vi "Engine-DI-Calibration.vi"(8 "error in (no error)":errorcluster, 9 "Inj Qtys DI-B":sgl[][](array[numeric]), 10 "Inj Qtys DI-A":sgl[][](array[numeric]), 11 "DCM DSI":refnum<class "DCM-DSI.lvclass">) -> (0 "error out":errorcluster, 3 "DCM DSI":refnum<class "DCM-DSI.lvclass">)   [LabVIEW 2016, in "DSI-RT.lvlib"]
uses:
  DSI-RT.lvlib
  Classes/DCM-DSI/DCM-DSI.lvclass
  Classes/DCM-DSI/Read DI-A Command.vi
  Classes/DCM-DSI/Read DI-B Command.vi
  Classes/DCM-DSI/Read Channels.vi
  Classes/DCM-DSI/Write DI-A Command.vi
  Classes/DCM-DSI/Write DI-B Command.vi
  <vilib>/addons/Software Calibration Management/xSCM/CalPoint.xnode
  <vilib>/addons/Software Calibration Management/xSCM/ni_scm.dll
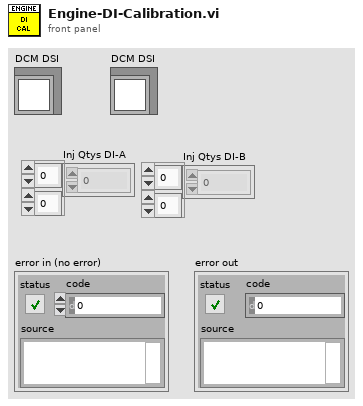
[diagram p1: front panel]
types:
  T1 = typedef "DCM - RT - DI.lvlib/Command.ctl" = cluster{"Mode":T2, "Digital Input":T3, "Default Profile Index":u8, "Cal Freq [Hz]":sgl, "Cal Duration [s]":sgl, "Cal Increment [s]":sgl, "Cal Pulses":u16, "TMP Command Sequence":T4[], "EPT TDC Offset [CAD]":sgl, "EPT Window Start [DBTDC]":sgl, "EPT Window End [DBTDC]":sgl, "EPT Angles":T5[], "EPT Skip Fire":bool, "EPT Skip Index":u8, "EPT Precharge Duration [s]":sgl, "EPT Precharge Profile Index":u8}
  T2 = typedef "DCM - FPGA - DI.lvlib/Mode.ctl" = enum8{"Off", "Direct", "Calibration", "Triggered Multi-Pulse", "Engine Position Tracking"}
  T3 = typedef "DCM - FPGA.lvlib/Digital Channel.ctl" = enum8{"Unused", "User OS", "Diff IO 1", "Diff IO 2", "Diff IO 3", "Diff IO 4", "Diff IO 5", "Diff IO 6", "Diff IO 7", "Diff IO 8", "Aux 1", "Aux 2", "Aux 3", "Aux 4", "Aux 5", "Aux 6", "Aux 7", "Aux 8", "Aux 9", "Aux 10", "Aux 11", "Aux 12", "Aux 13", "Aux 14", "Aux 15", "Aux 16"}
  T4 = typedef "DCM - RT - DI.lvlib/Command Sequence.ctl" = cluster{"Duration [s]":sgl, "Level":bool, "Run/Stop":bool, "Profile Index":u8}
  T5 = typedef "DCM - RT - DI.lvlib/Angle Control.ctl" = cluster{"Enable":bool, "Timing [DBTDC]":sgl, "Duration [s]":sgl, "Profile Index":u8}
  T6 = typedef "DCM-DSI.lvclass/Channel.ctl" = cluster{"Name":string, "Unit":string, "Value":sgl}
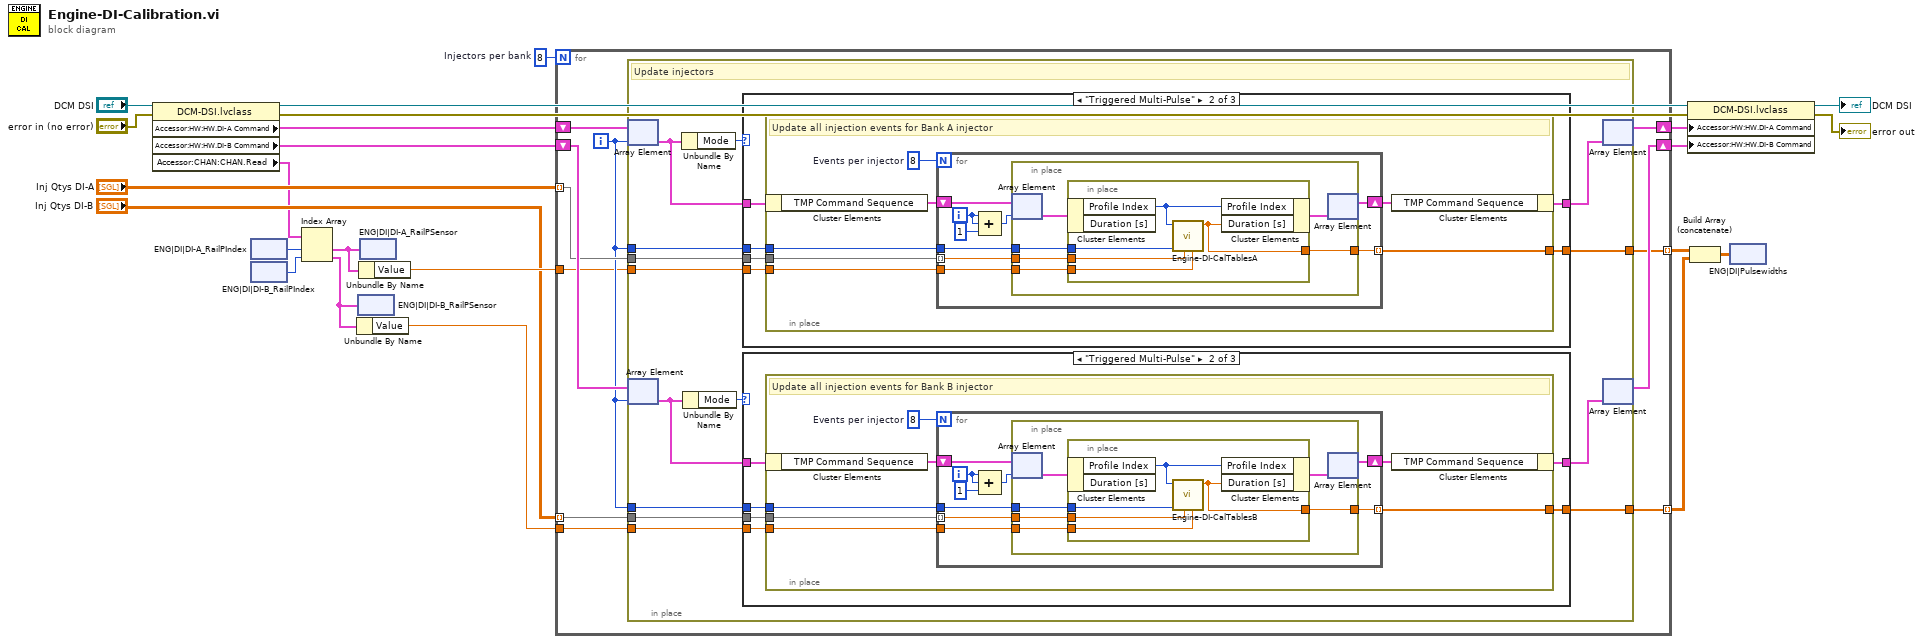
[diagram p0: block diagram]
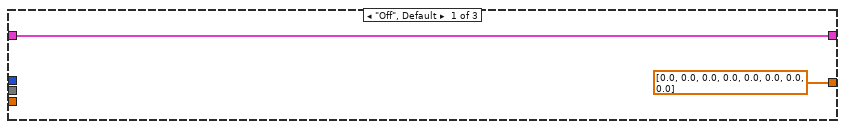
[diagram p2: hidden frame]
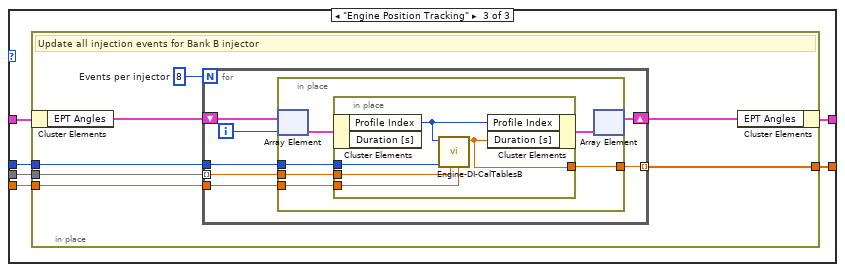
[diagram p3: hidden frame]
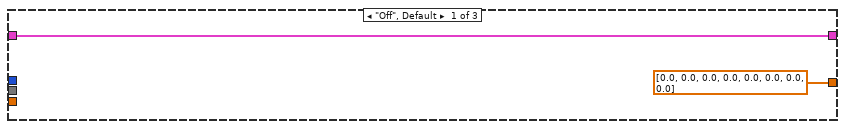
[diagram p4: hidden frame]
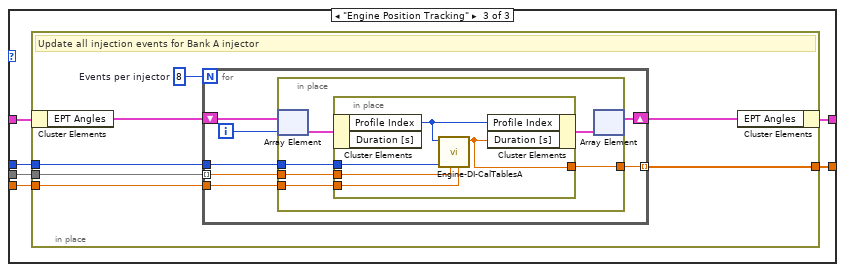
[diagram p5: hidden frame]
diagram:
  w22 = 8  # Injectors per bank
  n1 = property class="DCM-DSI.lvclass"(reference="DCM DSI", error in="error in (no error)") -> (reference out=w18:refnum<class "DCM-DSI.lvclass">, error out=w17:errorcluster, "Accessor:HW:HW.DI-A Command"=w9:T1[], "Accessor:HW:HW.DI-B Command"=w10:T1[], "Accessor:CHAN:CHAN.Read"=w5:T6[])
  n2 = xnode "ENG|DI|DI-A_RailPIndex"() -> ("Value"=w2:i32)
  n3 = xnode "ENG|DI|DI-B_RailPIndex"() -> ("Value"=w1:i32)
  n4 = Index Array(array=w5, index #1=w2, index #2=w1) -> (element #1=w3:T6, element #2=w4:T6)
  n5 = Unbundle By Name(w4) -> ("Value"=w21:sgl)
  n6 = xnode "ENG|DI|DI-B_RailPSensor"("Value"=w4) -> ()
  n7 = Unbundle By Name(w3) -> ("Value"=w23:sgl)
  n8 = xnode "ENG|DI|DI-A_RailPSensor"("Value"=w3) -> ()
  n9 = for {
    N: w22 -> [_]
    shift-right: [w33] -> w8
    shift-left: w9 -> [w34]
    tunnel: "Inj Qtys DI-A" -> [w30] mode=indexing
    tunnel: w21 -> [w28]
    shift-right: [w31] -> w7
    shift-left: w10 -> [w32]
    tunnel: "Inj Qtys DI-B" -> [w29] mode=indexing
    tunnel: w23 -> [w26]
    tunnel: [w25] -> w13 mode=indexing
    tunnel: [w24] -> w12 mode=indexing
    i -> [w27]
    n10 = in-place "Update Cylinders by IRQ call" {
      in-place-border: w29 -> [w39]
      in-place-border: w28 -> [w38]
      in-place-border: w27 -> [w40]
      in-place-border: w30 -> [w46]
      in-place-border: w26 -> [w47]
      in-place-border: w27 -> [w45]
      in-place-border: [w42] -> w25
      in-place-border: [w36] -> w24
      # "Update injectors"
      n11 = in-place-array #1(w34, w27) -> (w44:T1)
      n12 = in-place-array #2(w32, w27) -> (w37:T1)
      n13 = Unbundle By Name(w44) -> ("Mode"=w48:T2)
      n14 = Unbundle By Name(w37) -> ("Mode"=w41:T2)
      n15 = case shown="\"Triggered Multi-Pulse\"" w48 {
        tunnel: w44 -> [w116 w122 w155]
        tunnel: w45 -> [_ w121 w154]
        tunnel: w46 -> [_ w120 w153]
        tunnel: w47 -> [_ w119 w152]
        tunnel: [w116 w118 w151] -> w43
        tunnel: [sgl[] [0.0, 0.0, 0.0, 0.0, 0.0, 0.0, 0.0, 0.0] w117 w150] -> w42
        frame "Off", Default {
        }
        frame "Triggered Multi-Pulse" {
          n16 = in-place {
            in-place-border: w121 -> [w128]
            in-place-border: w120 -> [w127]
            in-place-border: w119 -> [w126]
            in-place-border: [w123] -> w117
            w124 = 8  # Events per injector
            # "Update all injection events for Bank A injector"
            n17 = in-place-cluster #3(w122) -> ("TMP Command Sequence"=w129:T4[])
            n18 = for {
              N: w124 -> [_]
              shift-right: [w137] -> w125
              shift-left: w129 -> [w138]
              tunnel: w128 -> [w136]
              tunnel: w127 -> [w135] mode=indexing
              tunnel: w126 -> [w134]
              tunnel: [w130] -> w123 mode=indexing
              i -> [w133]
              n19 = Compound Arithmetic op=ADD(w133, w133, 1 ("value")) -> (w131:i32)
              n20 = in-place {
                in-place-border: w136 -> [w142]
                in-place-border: w135 -> [w141]
                in-place-border: w134 -> [w140]
                in-place-border: [w139] -> w130
                n21 = in-place-array #4(w138, w131) -> (w144:T4)
                n22 = in-place {
                  in-place-border: w142 -> [w148]
                  in-place-border: w141 -> [w147]
                  in-place-border: w140 -> [w146]
                  in-place-border: [w145] -> w139
                  n23 = in-place-cluster #5(w144) -> ("Profile Index"=w149:u8)  [unwired: 1 out]
                  n24 = call "Engine-DI-CalTablesA.vi"("RailP [bar]"=w146, "InjQty [mm3/stroke]"=w147, "Injector"=w148, "Aux IDs"=w149) -> ("Durations [s]"=w145:sgl)  [unwired: 7 in]
                  n25 = in-place-cluster #5("Profile Index"=w149, "Duration [s]"=w145) -> (w143:T4)
                }
                n26 = in-place-array #4(w143) -> (w137:T4[])  [unwired: 1 out]
              }
            }
            n27 = in-place-cluster #3("TMP Command Sequence"=w125) -> (w118:T1)
          }
        }
        frame "Engine Position Tracking" {
          n28 = in-place {
            in-place-border: w154 -> [w161]
            in-place-border: w153 -> [w160]
            in-place-border: w152 -> [w159]
            in-place-border: [w156] -> w150
            w157 = 8  # Events per injector
            # "Update all injection events for Bank A injector"
            n29 = in-place-cluster #6(w155) -> ("EPT Angles"=w162:T5[])
            n30 = for {
              N: w157 -> [_]
              shift-right: [w168] -> w158
              shift-left: w162 -> [w169]
              tunnel: w161 -> [w167]
              tunnel: w160 -> [w166] mode=indexing
              tunnel: w159 -> [w165]
              tunnel: [w164] -> w156 mode=indexing
              i -> [w163]
              n31 = in-place {
                in-place-border: w167 -> [w173]
                in-place-border: w166 -> [w172]
                in-place-border: w165 -> [w171]
                in-place-border: [w170] -> w164
                n32 = in-place-array #7(w169, w163) -> (w175:T5)
                n33 = in-place {
                  in-place-border: w173 -> [w179]
                  in-place-border: w172 -> [w178]
                  in-place-border: w171 -> [w177]
                  in-place-border: [w176] -> w170
                  n34 = in-place-cluster #8(w175) -> ("Profile Index"=w180:u8)  [unwired: 1 out]
                  n35 = call "Engine-DI-CalTablesA.vi"("RailP [bar]"=w177, "InjQty [mm3/stroke]"=w178, "Injector"=w179, "Aux IDs"=w180) -> ("Durations [s]"=w176:sgl)  [unwired: 7 in]
                  n36 = in-place-cluster #8("Profile Index"=w180, "Duration [s]"=w176) -> (w174:T5)
                }
                n37 = in-place-array #7(w174) -> (w168:T5[])  [unwired: 1 out]
              }
            }
            n38 = in-place-cluster #6("EPT Angles"=w158) -> (w151:T1)
          }
        }
      }
      n39 = case shown="\"Triggered Multi-Pulse\"" w41 {
        tunnel: w37 -> [w50 w56 w89]
        tunnel: w40 -> [_ w55 w88]
        tunnel: w39 -> [_ w54 w87]
        tunnel: w38 -> [_ w53 w86]
        tunnel: [w50 w52 w85] -> w35
        tunnel: [sgl[] [0.0, 0.0, 0.0, 0.0, 0.0, 0.0, 0.0, 0.0] w51 w84] -> w36
        frame "Off", Default {
        }
        frame "Triggered Multi-Pulse" {
          n40 = in-place {
            in-place-border: w55 -> [w62]
            in-place-border: w54 -> [w61]
            in-place-border: w53 -> [w60]
            in-place-border: [w57] -> w51
            w58 = 8  # Events per injector
            # "Update all injection events for Bank B injector"
            n41 = in-place-cluster #9(w56) -> ("TMP Command Sequence"=w63:T4[])
            n42 = for {
              N: w58 -> [_]
              shift-right: [w71] -> w59
              shift-left: w63 -> [w72]
              tunnel: w62 -> [w70]
              tunnel: w61 -> [w69] mode=indexing
              tunnel: w60 -> [w68]
              tunnel: [w64] -> w57 mode=indexing
              i -> [w67]
              n43 = Compound Arithmetic op=ADD(w67, w67, 1 ("value")) -> (w65:i32)
              n44 = in-place {
                in-place-border: w70 -> [w76]
                in-place-border: w69 -> [w75]
                in-place-border: w68 -> [w74]
                in-place-border: [w73] -> w64
                n45 = in-place-array #10(w72, w65) -> (w78:T4)
                n46 = in-place {
                  in-place-border: w76 -> [w82]
                  in-place-border: w75 -> [w81]
                  in-place-border: w74 -> [w80]
                  in-place-border: [w79] -> w73
                  n47 = in-place-cluster #11(w78) -> ("Profile Index"=w83:u8)  [unwired: 1 out]
                  n48 = call "Engine-DI-CalTablesB.vi"("RailP [bar]"=w80, "InjQty [mm3/stroke]"=w81, "Injector"=w82, "Aux IDs"=w83) -> ("Durations [s]"=w79:sgl)  [unwired: 7 in]
                  n49 = in-place-cluster #11("Profile Index"=w83, "Duration [s]"=w79) -> (w77:T4)
                }
                n50 = in-place-array #10(w77) -> (w71:T4[])  [unwired: 1 out]
              }
            }
            n51 = in-place-cluster #9("TMP Command Sequence"=w59) -> (w52:T1)
          }
        }
        frame "Engine Position Tracking" {
          n52 = in-place {
            in-place-border: w88 -> [w95]
            in-place-border: w87 -> [w94]
            in-place-border: w86 -> [w93]
            in-place-border: [w90] -> w84
            w91 = 8  # Events per injector
            # "Update all injection events for Bank B injector"
            n53 = in-place-cluster #12(w89) -> ("EPT Angles"=w96:T5[])
            n54 = for {
              N: w91 -> [_]
              shift-right: [w102] -> w92
              shift-left: w96 -> [w103]
              tunnel: w95 -> [w101]
              tunnel: w94 -> [w100] mode=indexing
              tunnel: w93 -> [w99]
              tunnel: [w98] -> w90 mode=indexing
              i -> [w97]
              n55 = in-place {
                in-place-border: w101 -> [w107]
                in-place-border: w100 -> [w106]
                in-place-border: w99 -> [w105]
                in-place-border: [w104] -> w98
                n56 = in-place-array #13(w103, w97) -> (w109:T5)
                n57 = in-place {
                  in-place-border: w107 -> [w113]
                  in-place-border: w106 -> [w112]
                  in-place-border: w105 -> [w111]
                  in-place-border: [w110] -> w104
                  n58 = in-place-cluster #14(w109) -> ("Profile Index"=w114:u8)  [unwired: 1 out]
                  n59 = call "Engine-DI-CalTablesB.vi"("RailP [bar]"=w111, "InjQty [mm3/stroke]"=w112, "Injector"=w113, "Aux IDs"=w114) -> ("Durations [s]"=w110:sgl)  [unwired: 7 in]
                  n60 = in-place-cluster #14("Profile Index"=w114, "Duration [s]"=w110) -> (w108:T5)
                }
                n61 = in-place-array #13(w108) -> (w102:T5[])  [unwired: 1 out]
              }
            }
            n62 = in-place-cluster #12("EPT Angles"=w92) -> (w85:T1)
          }
        }
      }
      n63 = in-place-array #1(w43) -> (w33:T1[])  [unwired: 1 out]
      n64 = in-place-array #2(w35) -> (w31:T1[])  [unwired: 1 out]
    }
  }
  n65 = property class="DCM-DSI.lvclass"(reference=w18, error in=w17, "Accessor:HW:HW.DI-A Command"=w8, "Accessor:HW:HW.DI-B Command"=w7) -> (reference out=→"DCM DSI":refnum<class "DCM-DSI.lvclass">, error out=→"error out":errorcluster)
  n66 = Build Array (concatenate)(w13, w12) -> (w11:sgl[][])
  n67 = xnode "ENG|DI|Pulsewidths"("Value"=w11) -> ()
